vi "Read Configuration dict.vi"(8 "error in (no error)":errorcluster, 10 "Config Name":T1, 11 "Control in":refnum<class "Control-Server.lvclass">) -> (0 "error out":errorcluster, 2 "Config":refnum<class "Config.lvclass">, 3 "Control out":refnum<class "Control-Server.lvclass">)   [LabVIEW 2015, in "Control-Server.lvclass"]
uses:
  Control-Server.lvclass
  Config/config_names_def.ctl
  Config/Config.lvclass
  Control-Server.lvclass/Control-Server.ctl
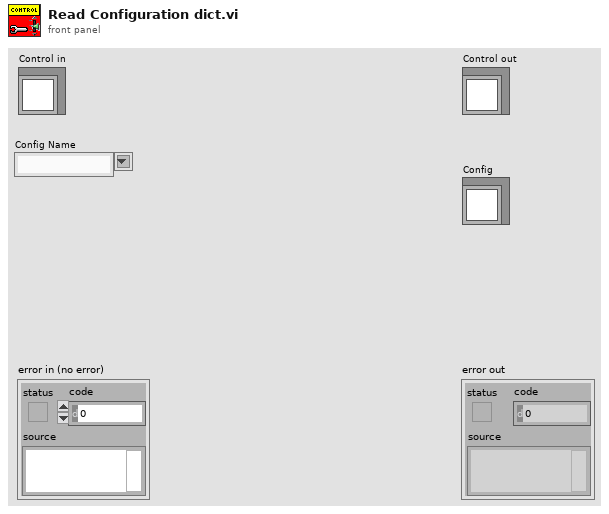
[diagram p1: front panel]
types:
  T1 = typedef "Config.lvclass/config_names_def.ctl" = string
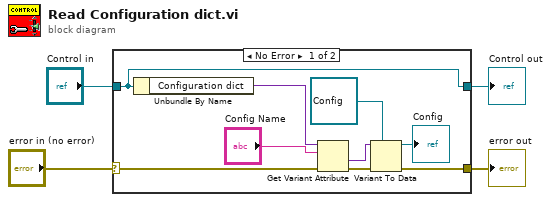
[diagram p0: block diagram]
diagram:
  n1 = case shown="No Error" "error in (no error)" {
    selector: "error in (no error)" -> [w8 w14]
    tunnel: [w7 w14] -> w3
    tunnel: [w13 w15] -> w1
    tunnel: "Control in" -> [w13 w15]
    frame No Error {
      n2 = Unbundle By Name(w13) -> ("Configuration dict"=w12:variant)
      n3 = Get Variant Attribute(Variant=w12, name="Config Name", error in=w8) -> (value=w10:variant, error out=w9:errorcluster)  [unwired: 1 in, 2 out]
      n4 = Variant To Data(error in=w9, type=refnum<class "Config.lvclass"> refnum ("Config.lvclass"), Variant=w10) -> (data=→"Config":refnum<class "Config.lvclass">, error out=w7:errorcluster)
    }
    frame Error {
    }
  }
  "error out" <- w3
  "Control out" <- w1
